vi "AutoIndexingTunnel.vi"() -> ()   [LabVIEW 2019]
uses:
  <vilib>/numeric/Random Number (Range) U64.vi
  <vilib>/numeric/sub_Random U32.vi
panel:
  out "Array 2":dbl[](array[numeric])
  out "Array":u64[](array[numeric])
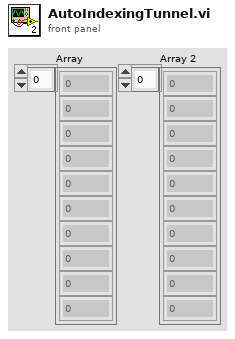
[diagram p1: front panel]
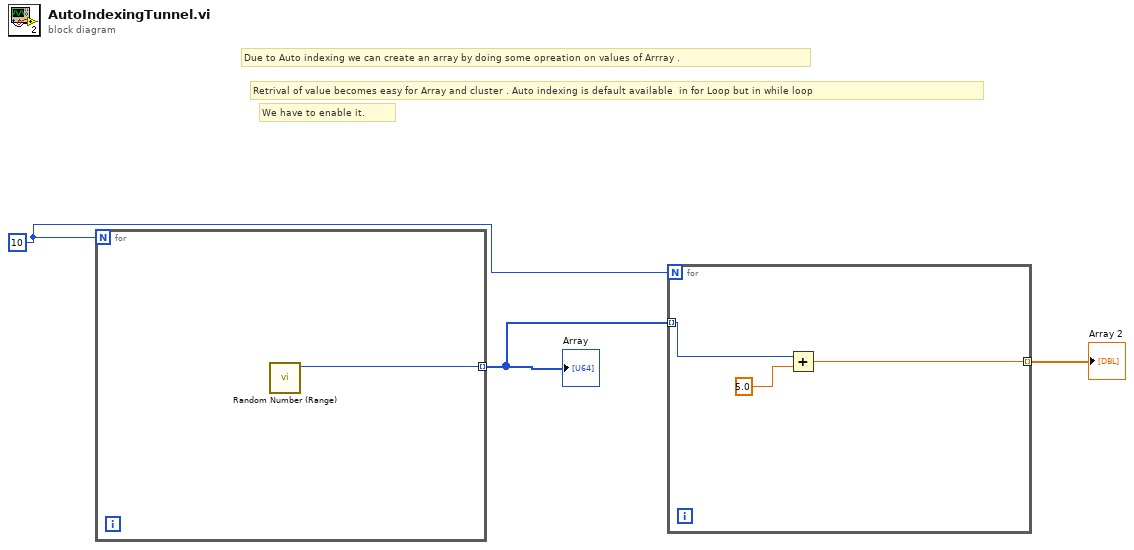
[diagram p0: block diagram]
diagram:
  w3 = 10
  # "We have to enable it."
  # "Retrival of value becomes easy for Array and cluster . Auto indexing is default available  in for Loop but in while loop"
  # "Due to Auto indexing we can create an array by doing some opreation on values of Arrray ."
  n1 = for {
    N: w3 -> [_]
    tunnel: [w4] -> w2 mode=indexing
    n2 = call-poly <vilib>:"Random Number (Range).vi"() -> ("number"=w4:u64)  [unwired: 11 in]
  }
  "Array" <- w2
  n3 = for {
    N: w3 -> [_]
    tunnel: w2 -> [w6] mode=indexing
    tunnel: [w5] -> w1 mode=indexing
    n4 = Add(x=w6, y=5.0) -> (x+y=w5:dbl)
  }
  "Array 2" <- w1
